vi "MCListBox Item Names to Object Names.vi"(7 "Item Names":string[][](array[string])) -> (3 "Object Names":string[](array[string]))   [LabVIEW 2019]
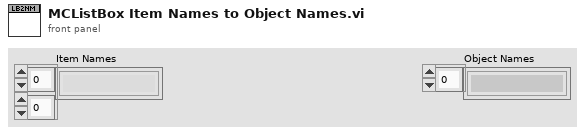
[diagram p1: front panel]
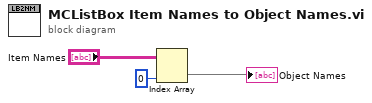
[diagram p0: block diagram]
diagram:
  n1 = Index Array(array="Item Names", index (col)=0 ("disabled index (col)")) -> (element=→"Object Names":string[])  [unwired: 1 in]
